vi "Log integration.vi"(8 "Error In":errorcluster, 9 "Min max":cluster{"Max":dbl, "Min":dbl}, 10 "Integration settings":T1={"Channel"="", "Output name"="", "Factor"=1.0, "Start time"=0.0, "Duration"=0.0} {"Duration" format="%#_6p"; "Start time" format="%#_6p"}, 11 "String":string) -> (0 "Error Out":errorcluster, 1 "Field":bool, 2 "Max":dbl, 3 "String out":string)   [LabVIEW 2015]
uses:
  Utilities/Controls/Integrate channel.ctl
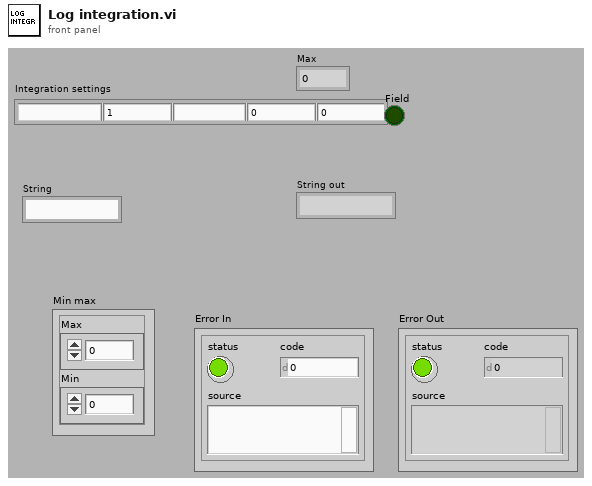
[diagram p1: front panel]
types:
  T1 = typedef "Integrate channel.ctl" = cluster{"Channel":string, "Output name":string, "Factor":dbl, "Start time":dbl, "Duration":dbl}
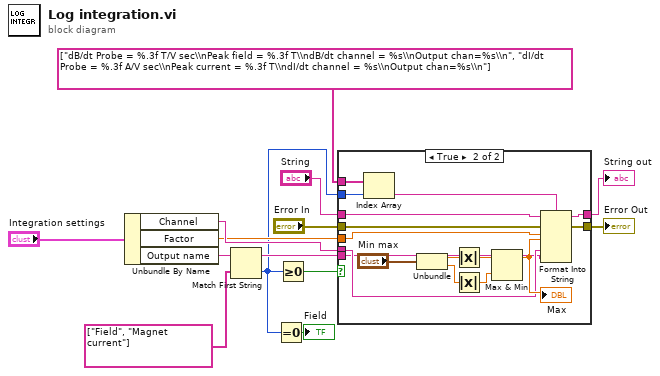
[diagram p0: block diagram]
diagram:
  n1 = Unbundle By Name("Integration settings") -> ("Channel"=w13:string, "Factor"=w12:dbl, "Output name"=w3:string)
  n2 = Match First String(2:string[] ["Field", "Magnet current"], 3:w3) -> (0:w2:i32)  [unwired: 1 out]
  n3 = Equal To 0?(x=w2) -> (x = 0?=→"Field":bool)
  n4 = Greater Or Equal To 0?(x=w2) -> (x >= 0?=w9:bool)
  n5 = case shown="True" w9 {
    tunnel: w13 -> [_ w30]
    tunnel: w12 -> [_ w29]
    tunnel: "String" -> [w15 w23]
    tunnel: [w15 w22] -> w7
    tunnel: string[] ["dB/dt Probe = %.3f T/V sec\\nPeak field = %.3f T\\ndB/dt channel = %s\\nOutput chan=%s\\n", "dI/dt Probe = %.3f A/V sec\\nPeak current = %.3f T\\ndI/dt channel = %s\\nOutput chan=%s\\n"] -> [_ w21]
    tunnel: w2 -> [_ w20]
    tunnel: "Error In" -> [w14 w18]
    tunnel: [w14 w17] -> w4
    tunnel: w3 -> [_ w16]
    frame False {
    }
    frame True {
      n6 = Index Array(array=w21, index=w20) -> (element=w19:string)
      n7 = Unbundle("Min max") -> ("Max"=w26:dbl, "Min"=w25:dbl)
      n8 = Absolute Value(x=w26) -> (abs(x)=w28:dbl)
      n9 = Absolute Value(x=w25) -> (abs(x)=w27:dbl)
      n10 = Max & Min(x=w28, y=w27) -> (max(x,y)=w31:dbl)  [unwired: 1 out]
      "Max" <- w31
      n11 = Format Into String(format string=w19, initial string=w23, error in=w18, w29, w31, w30, w16) -> (resulting string=w22:string, error out=w17:errorcluster)
    }
  }
  "String out" <- w7
  "Error Out" <- w4
